vi "测试项信息分解.vi"(8 "error in (no error)":errorcluster caption="错误输入（无错误）", 11 "当前产品检测信息":string) -> (0 "error out":errorcluster caption="错误输出", 3 "结果数组":string[](array[string]))   [LabVIEW 2017]
panel:
  out "数组":string[](array[string])
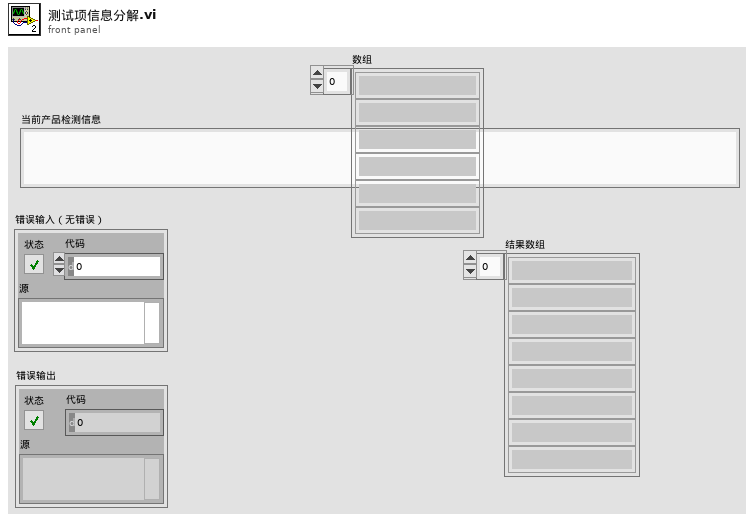
[diagram p1: front panel]
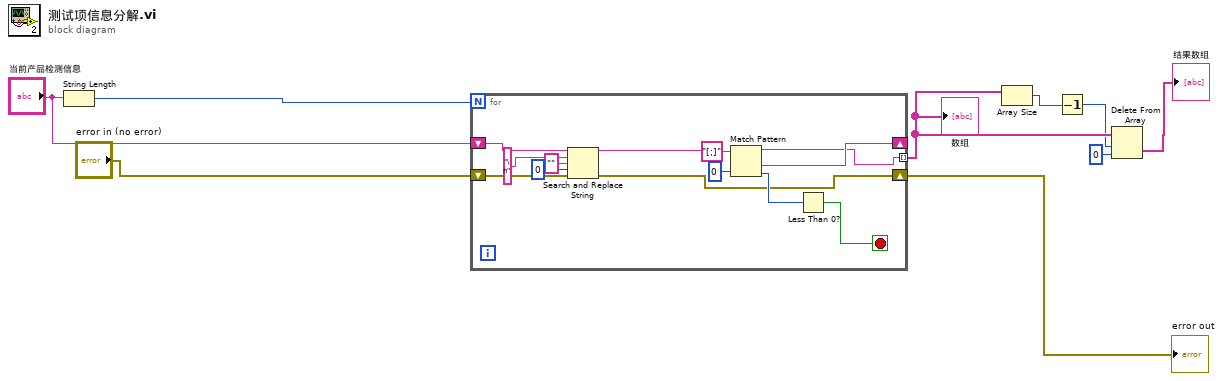
[diagram p0: block diagram]
diagram:
  n1 = String Length(string="当前产品检测信息") -> (length=w9:i32)
  n2 = for {
    N: w9 -> [_]
    shift-right: [w18] -> _
    shift-left: "当前产品检测信息" -> [w16]
    tunnel: [w17] -> w5 mode=indexing
    shift-right: [w11] -> w6
    shift-left: "error in (no error)" -> [w12]
    stop <- w19 stop-if-true
    n3 = Search and Replace String(input string=w16, search string="\n" ("搜索字符串"), replace string="" ("替换字符串(\"\")"), offset=0 ("偏移量(0)"), error in=w12) -> (result string=w15:string, error out=w11:errorcluster)  [unwired: 3 in, 2 out]
    n4 = Match Pattern(string=w15, regular expression="[;]" ("正则表达式"), offset (0)=0 ("偏移量(0)")) -> (before substring=w17:string, after substring=w18:string, offset past match=w20:i32)  [unwired: 1 out]
    n5 = Less Than 0?(x=w20) -> (x < 0?=w19:bool)
  }
  "error out" <- w6
  "数组" <- w5
  n6 = Array Size(array=w5) -> (size(s)=w4:i32)
  n7 = Decrement(x=w4) -> (x-1=w3:i32)
  n8 = Delete From Array(array=w5, length=w3, index=0 ("索引")) -> (deleted portion=→"结果数组":string[])  [unwired: 1 out]
